vi "Limit AO Amplitude.vi"(8 "error in (no error)":errorcluster, 10 "AO Amp Limit":dbl format="%.3p", 11 "Instrument.Lockin in":refnum<class "Instrument.Lockin.lvclass">) -> (0 "error out":errorcluster, 3 "Instrument.Lockin out":refnum<class "Instrument.Lockin.lvclass">)   [LabVIEW 2016, in "Instrument.Lockin.lvclass"]
uses:
  Instrument.Lockin.lvclass
  Instrument.Lockin.lvclass/Instrument.Lockin.ctl
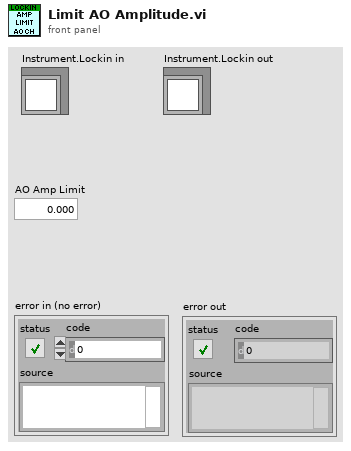
[diagram p1: front panel]
types:
  T1 = typedef "Lockin.DAQ.lvclass/AO-cluster.ctl" = T2[]
  T2 = typedef "Instrument.Lockin.UI.lvclass/AO Channel--Cluster.ctl" = cluster{"Channel":i32, "Amplitude":dbl, "Offset":dbl, "Frequency":dbl, "Phase":dbl, "Function":T3, "Sweeping?":bool, "REF.Ch 1":u16, "REF.Ch 2":u16}
  T3 = typedef "Lockin.DAQ.lvclass/Function-enum.ctl" = enum16{"Sine", "Triangle", "Square"}
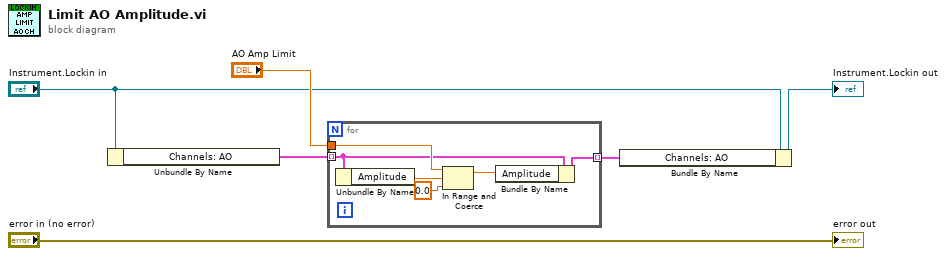
[diagram p0: block diagram]
diagram:
  n1 = Unbundle By Name("Instrument.Lockin in") -> ("Channels: AO"=w5:T1)
  n2 = for {
    tunnel: w5 -> [w9] mode=indexing
    tunnel: "AO Amp Limit" -> [w10]
    tunnel: [w7] -> w3 mode=indexing
    n3 = Unbundle By Name(w9) -> ("Amplitude"=w11:dbl)
    n4 = In Range and Coerce(upper limit=w10, x=w11, lower limit=0.0) -> (coerced(x)=w8:dbl)  [unwired: 1 out]
    n5 = Bundle By Name(cluster=w9, "Amplitude"=w8) -> (w7:T2)
  }
  n6 = Bundle By Name(cluster="Instrument.Lockin in", "Channels: AO"=w3) -> (→"Instrument.Lockin out":refnum<class "Instrument.Lockin.lvclass">)
  "error out" <- "error in (no error)"
